vi "report results.vi"(8 "error in":errorcluster, 10 "result":refnum<class "result.lvclass">, 11 "messenger reporter in":refnum<class "messenger reporter.lvclass">) -> (0 "error out":errorcluster, 3 "messenger reporter out":refnum<class "messenger reporter.lvclass">)   [LabVIEW 2014, in "messenger reporter.lvclass"]
uses:
  messenger reporter.lvclass
  result/result.lvclass
  result/result.lvclass/result.ctl
  <vilib>/drjdpowell/Messenging/Core Messages/Message/MSG.lvclass/MSG.ctl
  <vilib>/drjdpowell/Messenging/Core Messages/VarMessage/VariantMSG.lvclass/VariantMSG.ctl
  messenger reporter.lvclass/messenger reporter.ctl
  result/get data ID.vi
  result/get data.vi
  <vilib>/drjdpowell/Messenging/Core Messages/Message/Label Message.vi
  <vilib>/drjdpowell/Messenging/Core Messages/Message/Add Reply Address.vi
  <vilib>/drjdpowell/Messenging/Core Messages/VarMessage/VariantMSG.lvclass
  <vilib>/drjdpowell/Messenging/Core Messengers/Send/Send.lvclass
  <vilib>/drjdpowell/Messenging/Core Messages/MSG Library/SendMSG.lvlib
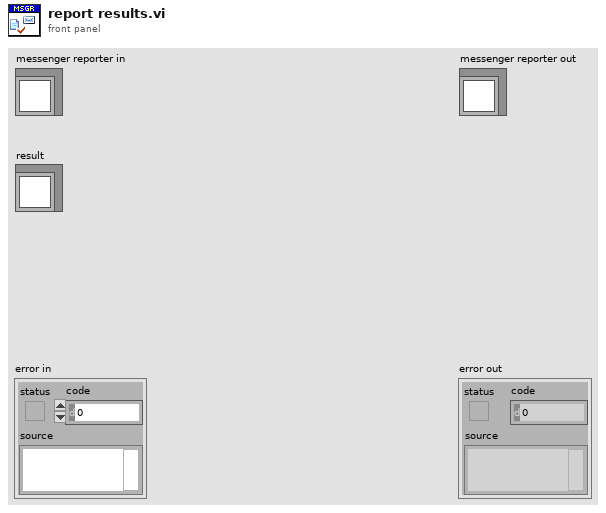
[diagram p1: front panel]
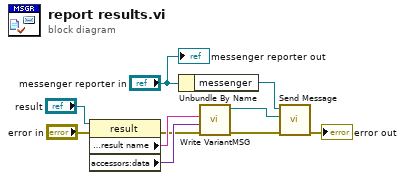
[diagram p0: block diagram]
diagram:
  n1 = property class="result"(reference="result", error in="error in") -> (error out=w5:errorcluster, "accessors:result name"=w6:string, "accessors:data"=w7:variant)  [unwired: 1 out]
  n2 = Unbundle By Name("messenger reporter in") -> ("messenger"=w2:refnum<class "Send.lvclass">)
  n3 = call <vilib>:"Write VariantMSG.vi"("error in (no error)"=w5, "Varient"=w7, "Label"=w6) -> ("error out"=w3:errorcluster, "Message"=w1:refnum<class "VariantMSG.lvclass">)  [unwired: 7 in]
  n4 = call <vilib>:"Send Message.vi"("error in (no error)"=w3, "Message"=w1, "Send In"=w2) -> ("error out"=→"error out":errorcluster)  [unwired: 7 in, 1 out]
  "messenger reporter out" <- "messenger reporter in"
